vi "GEOM_Sortby1coord.vi"(9 "amplifiers":T1[](array[typedef]) {"fliped" items=["none", "horizontal", "vertical"]; "type" items=["LL", "LR", "UL", "UR"]}, 10 "sort by":enum16{"x", "y"}(ring)) -> (1 "sorted amplifiers":T1[](array[typedef]) {"fliped" items=["none", "horizontal", "vertical"]; "type" items=["LL", "LR", "UL", "UR"]})   [LabVIEW 2016]
uses:
  GEOM_Amplifier.ctl
  GEOM_AmpType.ctl
  GEOM_ROI.ctl
  GEOM_Coords.ctl
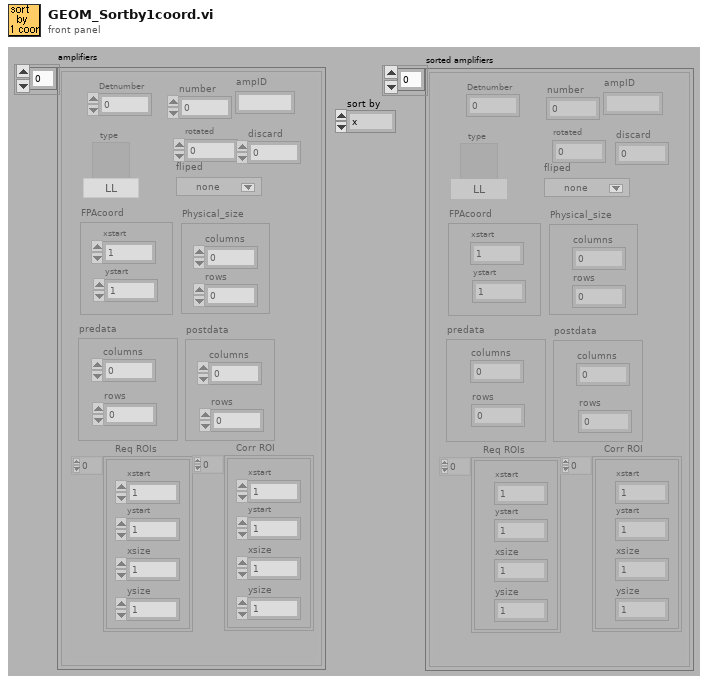
[diagram p1: front panel]
types:
  T1 = typedef "GEOM_Amplifier.ctl" = cluster{"number":i32, "type":T2, "rotated":i16, "fliped":u16, "FPAcoord":cluster{"xstart":i32, "ystart":i32}, "Physical_size":cluster{"columns":i32, "rows":i32}, "predata":cluster{"columns":i32, "rows":i32}, "postdata":cluster{"columns":i32, "rows":i32}, "Req ROIs":T3, "Corr ROI":T3, "Detnumber":i32, "ampID":string, "discard":i32}
  T2 = typedef "GEOM_AmpType.ctl" = u16
  T3 = typedef "GEOM_ROI.ctl" = T4[]
  T4 = typedef "GEOM_Coords.ctl" = cluster{"xstart":u32, "ystart":u32, "xsize":u32, "ysize":u32}
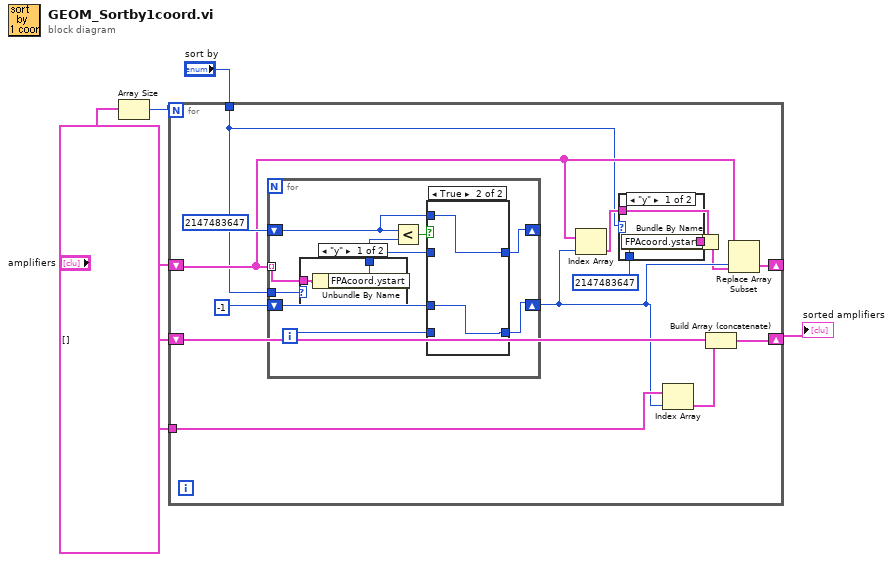
[diagram p0: block diagram]
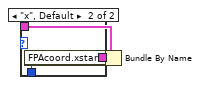
[diagram p2: hidden frame]
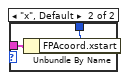
[diagram p3: hidden frame]
diagram:
  n1 = Array Size(array="amplifiers") -> (size(s)=w4:i32)
  n2 = for {
    N: w4 -> [_]
    shift-right: [w12] -> _
    shift-left: "amplifiers" -> [w10]
    shift-right: [w14] -> w5
    shift-left: T1[] [] -> [w13]
    tunnel: "amplifiers" -> [w16]
    tunnel: "sort by" -> [w6]
    n3 = for {
      shift-right: [w29] -> _
      shift-left: 2147483647 -> [w28]
      tunnel: w10 -> [w33] mode=indexing
      shift-right: [w27] -> w11
      shift-left: -1 -> [w26]
      tunnel: w6 -> [w25]
      i -> [w31]
      n4 = case shown="\"y\"" w25 {
        tunnel: w33 -> [w35 w37]
        tunnel: [w34 w36] -> w30
        frame "y" {
          n5 = Unbundle By Name(w35) -> ("FPAcoord.ystart"=w34:i32)
        }
        frame "x", Default {
          n6 = Unbundle By Name(w37) -> ("FPAcoord.xstart"=w36:i32)
        }
      }
      n7 = Less?(x=w28, y=w30) -> (x < y?=w32:bool)
      n8 = case shown="True" w32 {
        tunnel: w31 -> [w38 _]
        tunnel: w30 -> [w39 _]
        tunnel: [w39 w41] -> w29
        tunnel: w28 -> [_ w41]
        tunnel: [w38 w40] -> w27
        tunnel: w26 -> [_ w40]
        frame False {
        }
        frame True {
        }
      }
    }
    n9 = Index Array(array=w10, index=w11) -> (element=w9:T1)
    n10 = case shown="\"y\"" w6 {
      tunnel: w9 -> [w21 w24]
      tunnel: [w20 w23] -> w8
      tunnel: 2147483647 -> [w19 w22]
      frame "y" {
        n11 = Bundle By Name(cluster=w21, "FPAcoord.ystart"=w19) -> (w20:T1)
      }
      frame "x", Default {
        n12 = Bundle By Name(cluster=w24, "FPAcoord.xstart"=w22) -> (w23:T1)
      }
    }
    n13 = Index Array(array=w16, index=w11) -> (element=w15:T1)
    n14 = Build Array (concatenate)(w13, w15) -> (w14:T1[])
    n15 = Replace Array Subset(array=w10, new element=w8, index=w11) -> (w12:T1[])
  }
  "sorted amplifiers" <- w5
